vi "Parameter Set Write.vi"   [LabVIEW 2023, in "Cycler.lvclass"]
uses:
  Cycler.lvclass
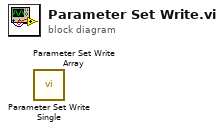
[diagram p0: block diagram]
diagram:
  n1 = call "Parameter Set Write Single.vi"() -> ()  [unwired: 12 in]
  n2 = call "Parameter Set Write Array.vi"() -> ()  [unwired: 10 in, 2 out]
